vi "cm2nm_transform_all_unvarified_spots.vi"(0 "Sample_Information":T3={"Sample Name/ID"="Granite 5 compare sessions 4 and 5", "Notes on Sample"="Sample was physically rotated relative to the coordinate system between sessions 4 and 5.", "Session_list"=[{"Instrument"=0, "Session_data_base"=path "/Documents and Settings/jannde/Desktop/Karens granite session 4 session5/Session 4/Session 4.xml", "Session Name/ID"="Session 4"}, {"Instrument"=0, "Session_data_base"=path "/Documents and Settings/jannde/Desktop/Karens granite session 4 session5/Session 5/Session 5.xml", "Session Name/ID"="Session 5"}, {"Instrument"=0, "Session_data_base"=path "/Documents and Settings/jannde/Desktop/Karens granite session 4 session5/Session 6/Session 6.xml", "Session Name/ID"="Session 6"}]}, 2 "Current Session Information IN":T5={"CollectionOfPoints"=[{"MetaDataFile"=path "", "X"=6.4684, "Y"=5.668, "Z"=0.0, "Group"=10, "Rotation"=0.0, "Fiducial"=TRUE, "Magnification"=0.0, "Working_Distance"=0.0, "Notes"="Enter notes about this spot here.", "Location Name/ID"="Fid1", "OtherRelatedDataFiles"=[], "Available"=FALSE}, {"MetaDataFile"=path "", "X"=6.7812, "Y"=-3.8607, "Z"=0.0, "Group"=10, "Rotation"=0.0, "Fiducial"=TRUE, "Magnification"=0.0, "Working_Distance"=0.0, "Notes"="Enter notes about this spot here.", "Location Name/ID"="Fid2", "OtherRelatedDataFiles"=[], "Available"=FALSE}, {"MetaDataFile"=path "", "X"=-3.5669, "Y"=-7.5774, "Z"=0.0, "Group"=10, "Rotation"=0.0, "Fiducial"=TRUE, "Magnification"=0.0, "Working_Distance"=0.0, "Notes"="Enter notes about this spot here.", "Location Name/ID"="Fid3", "OtherRelatedDataFiles"=[], "Available"=FALSE}, {"MetaDataFile"=path "", "X"=4.04214894226502, "Y"=-0.78740272281952, "Z"=0.0, "Group"=10, "Rotation"=0.0, "Fiducial"=FALSE, "Magnification"=0.0, "Working_Distance"=0.0, "Notes"="This is what we saw at the calculated coordinates for POI1. It's obviously not right! Look at images for calculated POI1.", "Location Name/ID"="POI1-calculated", "OtherRelatedDataFiles"=[], "Available"=FALSE}, {"MetaDataFile"=path "", "X"=0.4122, "Y"=-2.0241, "Z"=0.0, "Group"=0, "Rotation"=0.0, "Fiducial"=FALSE, "Magnification"=0.0, "Working_Distance"=0.0, "Notes"="These are the current coordinates of the real point", "Location Name/ID"="Actual POI1", "OtherRelatedDataFiles"=[], "Available"=FALSE}], "Instrument"=enum."Unknown", "CollectionFile"=path "/INL Macintosh/Users/timothymcjunkin/Documents/First_round_samples_FY2011_Test/Sample_9 Karens Granite/Karens granite session 4 session5 session6/Session 5/Session 5.xml", "Session Name/ID"="Session 5", "SessionNotes"="This is what we saw at the calculated coordinates for POI1. It's obviously not right! Look at images for calculated POI1."}, 12 "ReferenceSessionIndex":i32, 14 "TopLevelDataFilePath":path=path "/INL Macintosh/Users/timothymcjunkin/Documents/First_round_samples_FY2011_Test/Sample_9 Karens Granite/Karens granite session 4 session5 session6/Karens granite session4 session5 comparison.xml") -> (1 "Session Name/ID":string="Session 4", 4 "transfomration_matrices":T1, 5 "CurrentSessionOut":T6[](array[typedef])=[{"MetaDataFile"=path "", "X"=6.4684, "Y"=5.668, "Z"=0.0, "Group"=10, "Rotation"=0.0, "Fiducial"=TRUE, "Magnification"=0.0, "Working_Distance"=0.0, "Notes"="Enter notes about this spot here.", "Location Name/ID"="Fid1", "OtherRelatedDataFiles"=[], "Available"=FALSE}, {"MetaDataFile"=path "", "X"=6.7812, "Y"=-3.8607, "Z"=0.0, "Group"=10, "Rotation"=0.0, "Fiducial"=TRUE, "Magnification"=0.0, "Working_Distance"=0.0, "Notes"="Enter notes about this spot here.", "Location Name/ID"="Fid2", "OtherRelatedDataFiles"=[], "Available"=FALSE}, {"MetaDataFile"=path "", "X"=-3.5669, "Y"=-7.5774, "Z"=0.0, "Group"=10, "Rotation"=0.0, "Fiducial"=TRUE, "Magnification"=0.0, "Working_Distance"=0.0, "Notes"="Enter notes about this spot here.", "Location Name/ID"="Fid3", "OtherRelatedDataFiles"=[], "Available"=FALSE}, {"MetaDataFile"=path "", "X"=4.04214894226502, "Y"=-0.78740272281952, "Z"=0.0, "Group"=10, "Rotation"=0.0, "Fiducial"=FALSE, "Magnification"=0.0, "Working_Distance"=0.0, "Notes"="This is what we saw at the calculated coordinates for POI1. It's obviously not right! Look at images for calculated POI1.", "Location Name/ID"="POI1-calculated", "OtherRelatedDataFiles"=[], "Available"=FALSE}, {"MetaDataFile"=path "", "X"=0.4122, "Y"=-2.0241, "Z"=0.0, "Group"=0, "Rotation"=0.0, "Fiducial"=FALSE, "Magnification"=0.0, "Working_Distance"=0.0, "Notes"="These are the current coordinates of the real point", "Location Name/ID"="Actual POI1", "OtherRelatedDataFiles"=[], "Available"=FALSE}], 6 "FidcucialMetrics":cluster{"M1":dbl, "M2":dbl, "S1":dbl, "S2":dbl}, 7 "CurrentRefSessionIdx":i32, 8 "OK_num_fids?":bool, 9 "Current Session InformationOUT":T5={"CollectionOfPoints"=[{"MetaDataFile"=path "", "X"=6.4684, "Y"=5.668, "Z"=0.0, "Group"=10, "Rotation"=0.0, "Fiducial"=TRUE, "Magnification"=0.0, "Working_Distance"=0.0, "Notes"="Enter notes about this spot here.", "Location Name/ID"="Fid1", "OtherRelatedDataFiles"=[], "Available"=FALSE}, {"MetaDataFile"=path "", "X"=6.7812, "Y"=-3.8607, "Z"=0.0, "Group"=10, "Rotation"=0.0, "Fiducial"=TRUE, "Magnification"=0.0, "Working_Distance"=0.0, "Notes"="Enter notes about this spot here.", "Location Name/ID"="Fid2", "OtherRelatedDataFiles"=[], "Available"=FALSE}, {"MetaDataFile"=path "", "X"=-3.5669, "Y"=-7.5774, "Z"=0.0, "Group"=10, "Rotation"=0.0, "Fiducial"=TRUE, "Magnification"=0.0, "Working_Distance"=0.0, "Notes"="Enter notes about this spot here.", "Location Name/ID"="Fid3", "OtherRelatedDataFiles"=[], "Available"=FALSE}, {"MetaDataFile"=path "", "X"=4.04214894226502, "Y"=-0.78740272281952, "Z"=0.0, "Group"=10, "Rotation"=0.0, "Fiducial"=FALSE, "Magnification"=0.0, "Working_Distance"=0.0, "Notes"="This is what we saw at the calculated coordinates for POI1. It's obviously not right! Look at images for calculated POI1.", "Location Name/ID"="POI1-calculated", "OtherRelatedDataFiles"=[], "Available"=FALSE}, {"MetaDataFile"=path "", "X"=0.4122, "Y"=-2.0241, "Z"=0.0, "Group"=0, "Rotation"=0.0, "Fiducial"=FALSE, "Magnification"=0.0, "Working_Distance"=0.0, "Notes"="These are the current coordinates of the real point", "Location Name/ID"="Actual POI1", "OtherRelatedDataFiles"=[], "Available"=FALSE}, {"MetaDataFile"=path "", "X"=0.41202447787402247, "Y"=-2.022580250416809, "Z"=20.0, "Group"=10, "Rotation"=0.0, "Fiducial"=FALSE, "Magnification"=0.0, "Working_Distance"=0.0, "Notes"="Enter notes about this spot here.", "Location Name/ID"="POI1", "OtherRelatedDataFiles"=[], "Available"=FALSE}, {"MetaDataFile"=path "", "X"=-5.057894089920385, "Y"=8.260873627058263, "Z"=20.0, "Group"=10, "Rotation"=0.0, "Fiducial"=TRUE, "Magnification"=0.0, "Working_Distance"=0.0, "Notes"="Enter notes about this spot here.", "Location Name/ID"="Fid5", "OtherRelatedDataFiles"=[], "Available"=FALSE}, {"MetaDataFile"=path "", "X"=-9.447460259107727, "Y"=0.8548991441777762, "Z"=20.0, "Group"=10, "Rotation"=0.0, "Fiducial"=TRUE, "Magnification"=0.0, "Working_Distance"=0.0, "Notes"="Enter notes about this spot here.", "Location Name/ID"="Fid4", "OtherRelatedDataFiles"=[], "Available"=FALSE}], "Instrument"=enum."Unknown", "CollectionFile"=path "/INL Macintosh/Users/timothymcjunkin/Documents/First_round_samples_FY2011_Test/Sample_9 Karens Granite/Karens granite session 4 session5 session6/Session 5/Session 5.xml", "Session Name/ID"="Session 5", "SessionNotes"="This is what we saw at the calculated coordinates for POI1. It's obviously not right! Look at images for calculated POI1."}, 10 "ReferenceSet":T5={"CollectionOfPoints"=[{"MetaDataFile"=path "", "X"=-7.9056, "Y"=2.6841, "Z"=0.0, "Group"=10, "Rotation"=0.0, "Fiducial"=TRUE, "Magnification"=0.0, "Working_Distance"=0.0, "Notes"="Enter notes about this spot here.", "Location Name/ID"="Fid1", "OtherRelatedDataFiles"=[], "Available"=FALSE}, {"MetaDataFile"=path "", "X"=-0.1023, "Y"=8.1499, "Z"=0.0, "Group"=10, "Rotation"=0.0, "Fiducial"=TRUE, "Magnification"=0.0, "Working_Distance"=0.0, "Notes"="Enter notes about this spot here.", "Location Name/ID"="Fid2", "OtherRelatedDataFiles"=[], "Available"=FALSE}, {"MetaDataFile"=path "", "X"=8.6459, "Y"=1.4833, "Z"=0.0, "Group"=10, "Rotation"=0.0, "Fiducial"=TRUE, "Magnification"=0.0, "Working_Distance"=0.0, "Notes"="Enter notes about this spot here.", "Location Name/ID"="Fid3", "OtherRelatedDataFiles"=[], "Available"=FALSE}, {"MetaDataFile"=path "", "X"=4.7936, "Y"=-8.0627, "Z"=0.0, "Group"=10, "Rotation"=0.0, "Fiducial"=TRUE, "Magnification"=0.0, "Working_Distance"=0.0, "Notes"="Enter notes about this spot here.", "Location Name/ID"="Fid4", "OtherRelatedDataFiles"=[], "Available"=FALSE}, {"MetaDataFile"=path "", "X"=-3.7954, "Y"=-8.4178, "Z"=0.0, "Group"=10, "Rotation"=0.0, "Fiducial"=TRUE, "Magnification"=0.0, "Working_Distance"=0.0, "Notes"="Enter notes about this spot here.", "Location Name/ID"="Fid5", "OtherRelatedDataFiles"=[], "Available"=FALSE}, {"MetaDataFile"=path "", "X"=1.8297, "Y"=1.7939, "Z"=0.0, "Group"=10, "Rotation"=0.0, "Fiducial"=FALSE, "Magnification"=0.0, "Working_Distance"=0.0, "Notes"="Enter notes about this spot here.", "Location Name/ID"="POI1", "OtherRelatedDataFiles"=[], "Available"=FALSE}], "Instrument"=enum."Unknown", "CollectionFile"=path "/INL Macintosh/Users/timothymcjunkin/Documents/First_round_samples_FY2011_Test/Sample_9 Karens Granite/Karens granite session 4 session5 session6/Session 4/Session 4.xml", "Session Name/ID"="Session 4", "SessionNotes"="Repeats earlier session 4 data"}, 11 "Array":bool[](array[boolean])=[TRUE, TRUE, TRUE, FALSE, FALSE, FALSE], 13 "Best_fit_and_name_match.":bool, 15 "PairedFiducialNames":T4(array[cluster])=[{"Location Name/ID"="Fid1", "Location Name/ID"="Fid1"}, {"Location Name/ID"="Fid2", "Location Name/ID"="Fid2"}, {"Location Name/ID"="Fid3", "Location Name/ID"="Fid3"}])   [LabVIEW 2011]
doc: "This calls the routine to calculate the transformation matrix for a chosen session. That routine will actually search backwards from that session until it finds one with enough matching fiducials. From there the points are matched and replaced or added in the current session collection of points. Group number may be changed to indicate it is a calculated point. \n\nThe software loops through the points and compares the names to those already in this session. If they are in the session and were previously calculated the new calculation replaces the old one. If they are calculated and not currently there they are appended to the list. If they are entered they are not changed. \n\nThis was done to have all the calculated spots ready for the user or to be there if they were to be calculated forward to future sesions."
uses:
  cm2nm_sample_set.ctl
  cm2nm_coordinate_information_v2.ctl
  Instrument_type_enum_v2.ctl
  transformMatrix.ctl
  <vilib>/Analysis/Matrix/Datatypes/RealMatrix.ctl
  <vilib>/Analysis/Matrix/NI_Matrix.lvlib
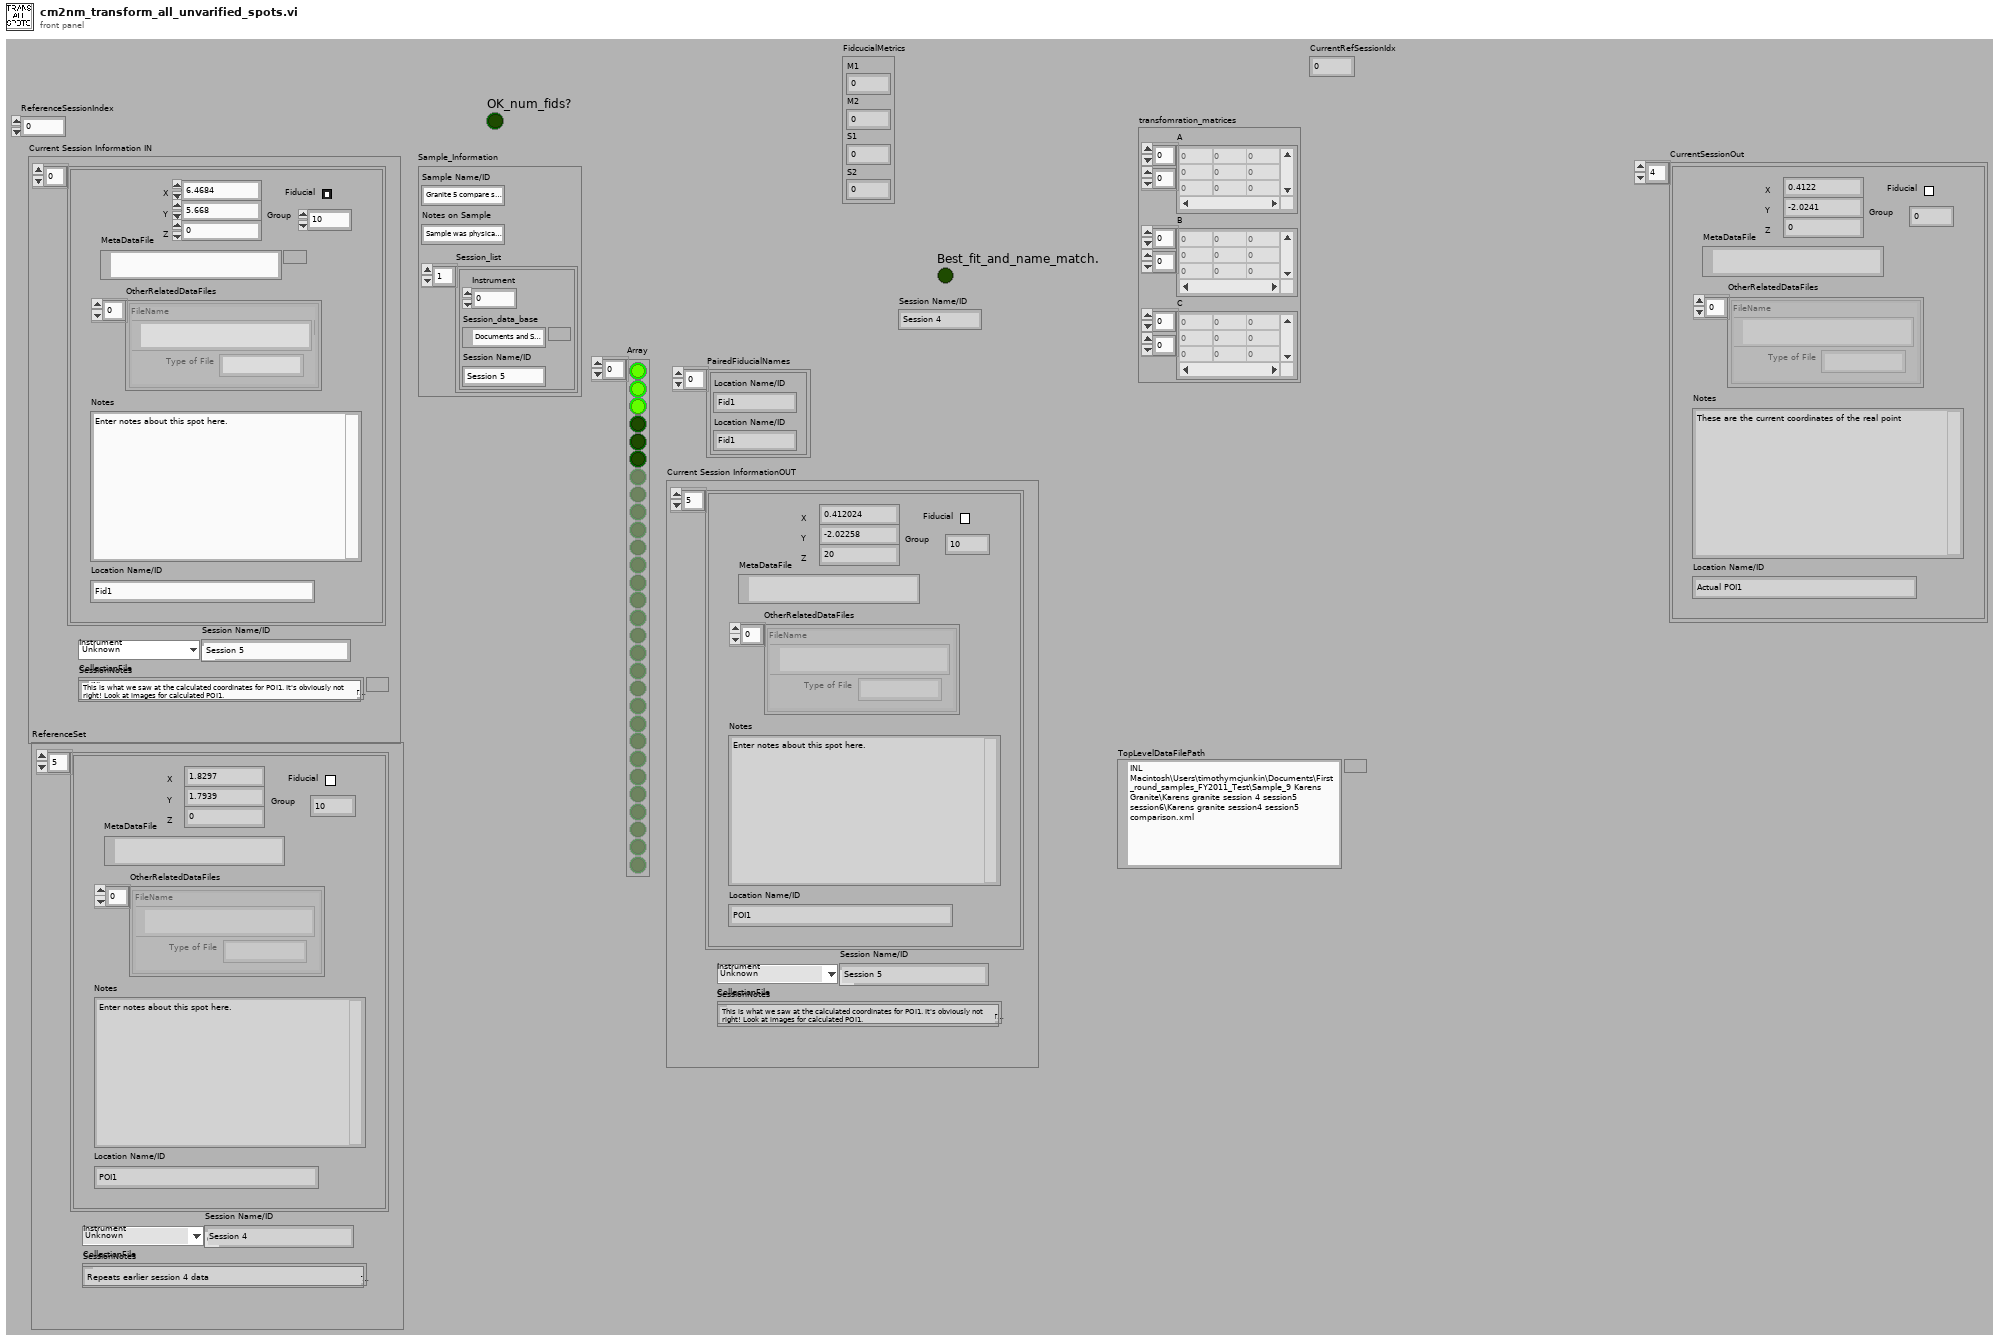
[diagram p1: front panel]
types:
  T1 = typedef "transformMatrix.ctl" = cluster{"A":T2, "B":T2, "C":T2}
  T2 = typedef "NI_Matrix.lvlib/RealMatrix.ctl" = dbl[][]
  T3 = cluster{"Sample Name/ID":string, "Notes on Sample":string, "Session_list":cluster{"Instrument":u16, "Session_data_base":path, "Session Name/ID":string}[]}
  T4 = cluster{"Location Name/ID":string, "Location Name/ID":string}[]
  T5 = typedef "cm2nm_sample_set.ctl" = cluster{"CollectionOfPoints":T6[], "Instrument":T7, "CollectionFile":path, "Session Name/ID":string, "SessionNotes":string}
  T6 = typedef "cm2nm_coordinate_information_v2.ctl" = cluster{"MetaDataFile":path, "X":dbl, "Y":dbl, "Z":dbl, "Group":i32, "Rotation":dbl[unit], "Fiducial":bool, "Magnification":dbl, "Working_Distance":dbl, "Notes":string, "Location Name/ID":string, "OtherRelatedDataFiles":cluster{"Type of File":string, "FileName":path}[], "Available":bool}
  T7 = typedef "Instrument_type_enum_v2.ctl" = enum16{"Unknown", "Philips FEI SEM IRC", "JEOL 7000F EML_MFC", "MXRD MFC", "JEOL_EPMA"}
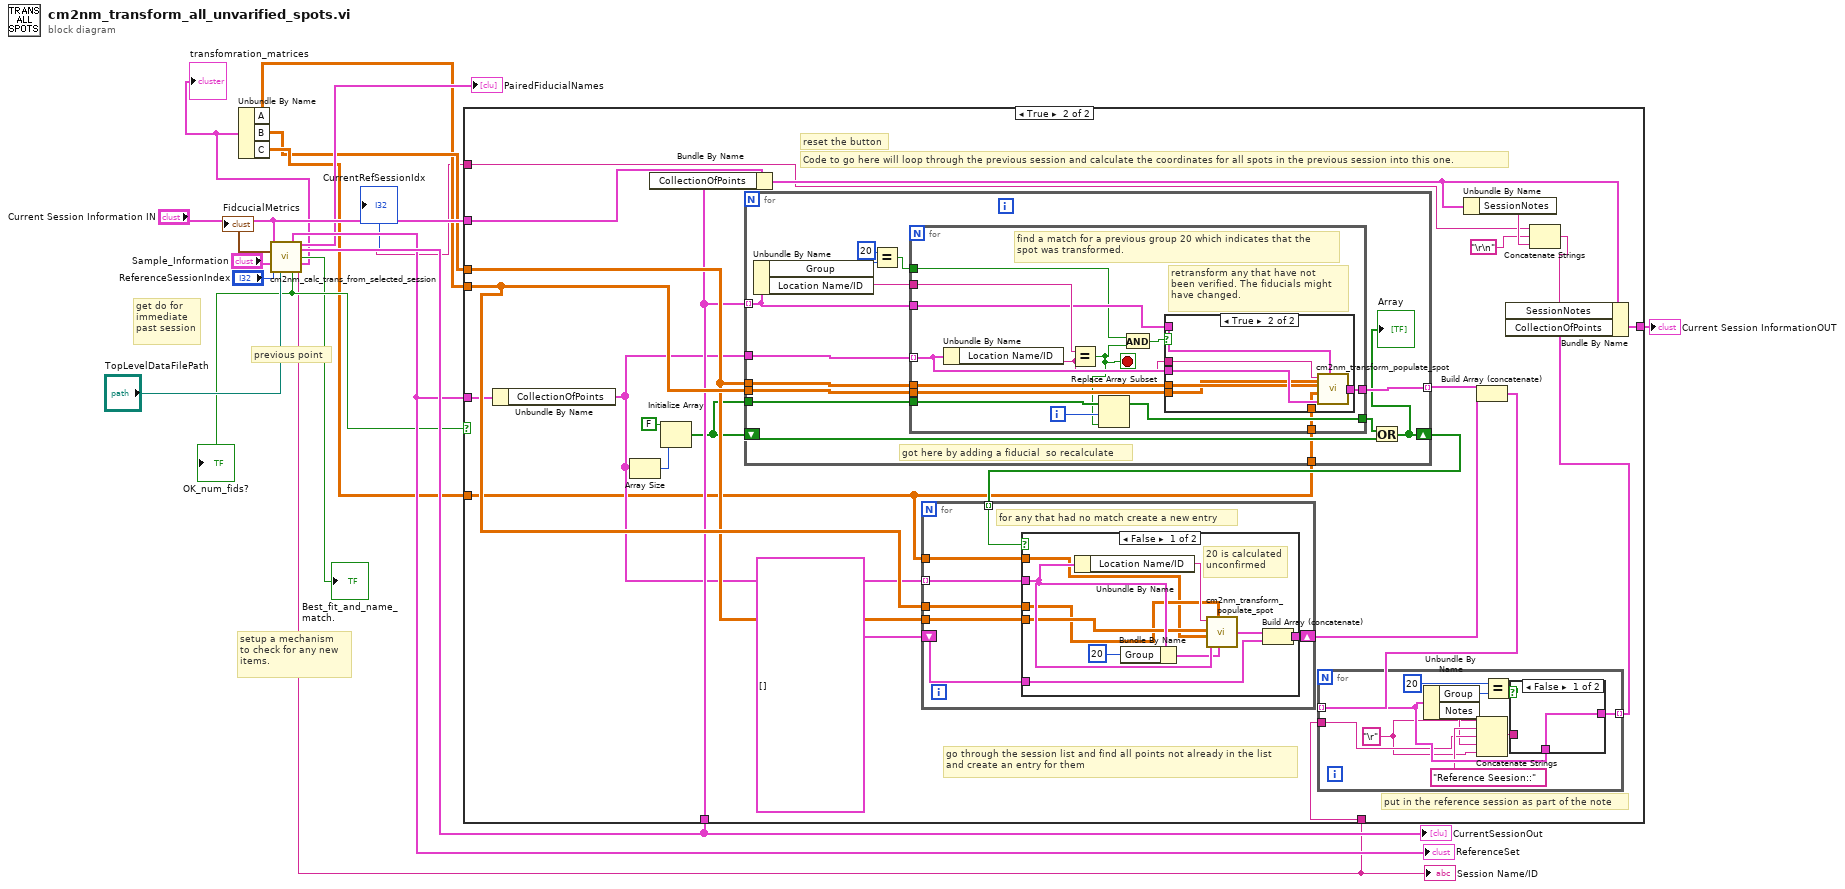
[diagram p0: block diagram]
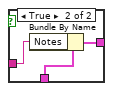
[diagram p3: hidden frame]
diagram:
  # "setup a mechanism\nto check for any new\nitems."
  # "previous point"
  # "get do for\nimmediate\npast session"
  n1 = call "cm2nm_calc_trans_from_selected_session.vi"("Current Session Information"="Current Session Information IN", "Sample_Information"="Sample_Information", "SessionIndex"="ReferenceSessionIndex", "TopLevelDataFilePath"="TopLevelDataFilePath") -> ("CurrentRefSessionIdx"=→"CurrentRefSessionIdx":i32, "CurrentSessionOut"=w17:T6[], "ReferenceSession"=w15:T5, "PairedFiducialNames"=→"PairedFiducialNames":T4, "FidcucialMetrics"=→"FidcucialMetrics":cluster{"M1":dbl, "M2":dbl, "S1":dbl, "S2":dbl}, "Matrices_in_text"=w2:string, "Best_fit_and_name_match."=→"Best_fit_and_name_match.":bool, "transfrom_matrices"=w3:T1, "OK_num_fids?"=w10:bool, "ReferenceSession Name/ID"=w7:string)  [unwired: 1 in, 1 out]
  "CurrentSessionOut" <- w17
  "ReferenceSet" <- w15
  "Session Name/ID" <- w7
  "OK_num_fids?" <- w10
  "transfomration_matrices" <- w3
  n2 = Unbundle By Name(w3) -> ("A"=w4:T2, "B"=w5:T2, "C"=w6:T2)
  n3 = case shown="True" w10 {
    tunnel: w4 -> [_ w42]
    tunnel: w5 -> [_ w41]
    tunnel: [w19 w40] -> w18
    tunnel: w17 -> [_ w38]
    tunnel: "Current Session Information IN" -> [w19 w37]
    tunnel: w15 -> [_ w36]
    tunnel: w6 -> [_ w28]
    tunnel: w7 -> [_ w26]
    tunnel: w2 -> [_ w22]
    frame False {
      # "if not correct number of fiducials don't do anything."
    }
    frame True {
      # "put in the reference session as part of the note"
      # "go through the session list and find all points not already in the list\nand create an entry for them"
      # "Code to go here will loop through the previous session and calculate the coordinates for all spots in the previous session into this one."
      # "reset the button"
      n4 = Unbundle By Name(w36) -> ("CollectionOfPoints"=w32:T6[])
      n5 = Array Size(array=w32) -> (size(s)=w30:i32)
      n6 = Bundle By Name(cluster=w37, "CollectionOfPoints"=w38) -> (w24:T5)
      n7 = Initialize Array(FALSE ("x = y?"), w30) -> (w29:bool[])
      n8 = for {
        tunnel: w32 -> [w88]
        tunnel: w38 -> [w87] mode=indexing
        tunnel: [w82] -> w34 mode=indexing
        shift-right: [w76] -> w39
        shift-left: w29 -> [w81]
        tunnel: w41 -> [w80]
        tunnel: w42 -> [w79]
        tunnel: w29 -> [w78]
        tunnel: w28 -> [w75]
        # "got here by adding a fiducial  so recalculate"
        n9 = Unbundle By Name(w87) -> ("Group"=w85:i32, "Location Name/ID"=w86:string)
        n10 = Equal?(x=20, y=w85) -> (x = y?=w83:bool)
        n11 = for {
          tunnel: w88 -> [w102] mode=indexing
          tunnel: w87 -> [w99]
          tunnel: w86 -> [w101]
          tunnel: w83 -> [w96]
          tunnel: [w100] -> w82
          tunnel: w80 -> [w98]
          tunnel: w79 -> [w97]
          tunnel: w78 -> [w93]
          tunnel: [w91] -> w77
          tunnel: w75 -> [w89]
          i -> [w94]
          stop <- w90 stop-if-true
          # "retransform any that have not\nbeen verified. The fiducials might\nhave changed."
          # "find a match for a previous group 20 which indicates that the\nspot was transformed."
          n12 = Unbundle By Name(w102) -> ("Location Name/ID"=w95:string)
          n13 = Equal?(x=w101, y=w95) -> (x = y?=w90:bool)
          n14 = Replace Array Subset(array=w93, new element=w90, index=w94) -> (w91:bool[])
          n15 = And(x=w96, y=w90) -> (x .and. y?=w92:bool)
          n16 = case shown="True" w92 {
            tunnel: w102 -> [_ w110]
            tunnel: w99 -> [w103 w109]
            tunnel: [w103 w108] -> w100
            tunnel: w98 -> [_ w107]
            tunnel: w97 -> [_ w106]
            tunnel: w95 -> [_ w105]
            tunnel: w89 -> [_ w104]
            frame False {
              # "if it is not equal or not group of \n20 then pass through"
            }
            frame True {
              n17 = call "cm2nm_transform_populate_spot.vi"("NewPointIn"=w109, "A - Transformation Matrix"=w106, "Previous Session Spot"=w110, "C"=w104, "B - vector offset"=w107, "Spot_ID"=w105) -> ("NewPointOut"=w108:T6)
            }
          }
        }
        n18 = Or(x=w77, y=w81) -> (x .or. y?=w76:bool[])
        "Array" <- w76
      }
      n19 = for {
        tunnel: w39 -> [w63] mode=indexing
        tunnel: w32 -> [w62] mode=indexing
        shift-right: [w60] -> w35
        shift-left: T6[] [] -> [w61]
        tunnel: w41 -> [w59]
        tunnel: w42 -> [w58]
        tunnel: w28 -> [w57]
        # "for any that had no match create a new entry"
        n20 = case shown="False" w63 {
          tunnel: w62 -> [w72 _]
          tunnel: w61 -> [w68 w74]
          tunnel: [w67 w74] -> w60
          tunnel: w59 -> [w66 _]
          tunnel: w58 -> [w65 _]
          tunnel: w57 -> [w64 _]
          frame False {
            # "20 is calculated\nunconfirmed"
            n21 = Unbundle By Name(w72) -> ("Location Name/ID"=w73:string)
            n22 = Bundle By Name(cluster=w72, "Group"=20) -> (w70:T6)
            n23 = call "cm2nm_transform_populate_spot.vi"("NewPointIn"=w70, "A - Transformation Matrix"=w65, "Previous Session Spot"=w72, "C"=w64, "B - vector offset"=w66, "Spot_ID"=w73) -> ("NewPointOut"=w69:T6)
            n24 = Build Array (concatenate)(w69, w68) -> (w67:T6[])
          }
          frame True {
          }
        }
      }
      n25 = Unbundle By Name(w24) -> ("SessionNotes"=w23:string)
      n26 = Build Array (concatenate)(w34, w35) -> (w27:T6[])
      n27 = for {
        tunnel: w27 -> [w49] mode=indexing
        tunnel: w26 -> [w47]
        tunnel: [w45] -> w25 mode=indexing
        w43 = "\r" ("string")
        n28 = Unbundle By Name(w49) -> ("Group"=w52:i32, "Notes"=w44:string)
        n29 = Concatenate Strings(w43, "Reference Seesion::" ("string"), w47, w44, w43) -> (w46:string)
        n30 = Equal?(x=20, y=w52) -> (x = y?=w50:bool)
        n31 = case shown="False" w50 {
          tunnel: w49 -> [w53 w56]
          tunnel: w46 -> [_ w55]
          tunnel: [w53 w54] -> w45
          frame False {
          }
          frame True {
            n32 = Bundle By Name(cluster=w56, "Notes"=w55) -> (w54:T6)
          }
        }
      }
      n33 = Concatenate Strings(w22, "\r\n", w23) -> (w20:string)
      n34 = Bundle By Name(cluster=w24, "SessionNotes"=w20, "CollectionOfPoints"=w25) -> (w40:T5)
    }
  }
  "Current Session InformationOUT" <- w18
